vi "TxRx SingleBoard (SubVI).vi"(0 "VISA Refnum in":refnum<visa-resource-name>, 2 "DataMessage Tx":T2={"Send Debug"="", "idx"=0, "DataType"=enum."Int", "Cmd id"=200, "Get/Set"=enum."Set"}, 3 "Tx":refnum<vi>, 4 "Rx":refnum<vi>, 5 "error in (no error)":errorcluster, 6 "Tx semaphore":T1, 8 "Rx semaphore":T1) -> (12 "output array":u8[](array[numeric]) format="%.0x", 14 "VISA Refnum out":refnum<visa-resource-name>, 15 "RxMessage":u8[](array[numeric]) format="%x", 16 "DataReceived?":bool, 17 "CRC":bool, 18 "Get/Set":enum8{"Set", "Get"}(ring), 19 "error out":errorcluster)   [LabVIEW 2017]
panel:
  out "TxMsg":u8[](array[numeric]) format="%.0x"
  # "Value"
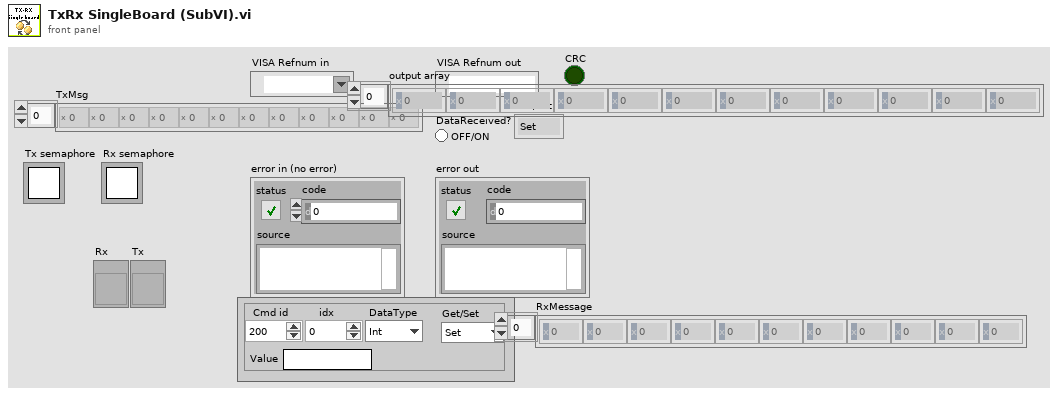
[diagram p1: front panel]
types:
  T1 = typedef "Semaphore RefNum" = refnum<k1>
  T2 = cluster{"Send Debug":string, "idx":u16, "DataType":enum8{"Int", " float"}, "Cmd id":u16, "Get/Set":enum8{"Set", "Get"}}
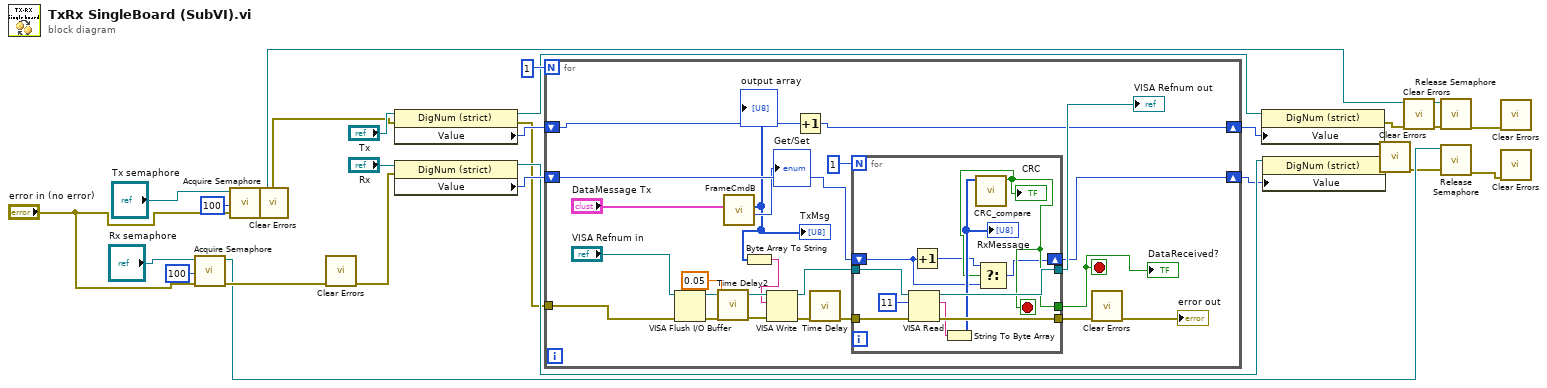
[diagram p0: block diagram]
diagram:
  n1 = call <vilib>:"Acquire Semaphore.vi"("error in (no error)"="error in (no error)", "ms timeout (-1)"=100, "semaphore"="Rx semaphore") -> ("error out"=w12:errorcluster, "semaphore out"=w8:T1)  [unwired: 2 in, 1 out]
  n2 = call <vilib>:"Acquire Semaphore.vi"("error in (no error)"="error in (no error)", "ms timeout (-1)"=100, "semaphore"="Tx semaphore") -> ("error out"=w16:errorcluster, "semaphore out"=w11:T1)  [unwired: 2 in, 1 out]
  n3 = call <vilib>:"Clear Errors.vi"("error in (no error)"=w16) -> ("error out"=w2:errorcluster)  [unwired: 5 in, 1 out]
  n4 = call <vilib>:"Clear Errors.vi"("error in (no error)"=w12) -> ("error out"=w1:errorcluster)  [unwired: 5 in, 1 out]
  n5 = property class="DigNum (strict)"(reference="Tx", error in=w2) -> (reference out=w22:refnum<vi>, error out=w15:errorcluster, "Value"=w23:u64)
  n6 = property class="DigNum (strict)"(reference="Rx", error in=w1) -> (reference out=w21:refnum<vi>, "Value"=w24:u64)  [unwired: 1 out]
  n7 = for {
    N: 1 -> [_]
    shift-right: [w36] -> w20
    shift-left: w23 -> [w38]
    shift-right: [w35] -> w19
    shift-left: w24 -> [w37]
    tunnel: w15 -> [w34]
    stop <- w41 stop-if-true
    n8 = VISA Flush I/O Buffer(VISA resource name="VISA Refnum in", error in (no error)=w34) -> (VISA resource name out=w44:refnum<visa-resource-name>, error out=w33:errorcluster)  [unwired: 1 in]
    n9 = call "Time Delay2"("error in (no error)"=w33, "Delay Time (s)"=0.05) -> ("error out"=w32:errorcluster)  [unwired: 9 in]
    n10 = call "FrameCmdB.vi"("DataMessage"="DataMessage Tx") -> ("Get/Set"=→"Get/Set":enum8{"Set", "Get"}, "output array"=w29:u8[])  [unwired: 7 in, 2 out]
    "TxMsg" <- w29
    "output array" <- w29
    n11 = Byte Array To String(unsigned byte array=w29) -> (string=w28:string)
    n12 = VISA Write(VISA resource name=w44, write buffer=w28, error in (no error)=w32) -> (VISA resource name out=w45:refnum<visa-resource-name>, error out=w48:errorcluster)  [unwired: 1 out]
    n13 = Increment(x=w38) -> (x+1=w36:u64)
    n14 = call "Time Delay"("error in (no error)"=w48) -> ("error out"=w49:errorcluster)  [unwired: 10 in]
    n15 = for {
      N: 1 -> [_]
      tunnel: [w53] -> w41
      tunnel: w49 -> [w60]
      tunnel: [w58] -> w46
      tunnel: w45 -> [w56]
      tunnel: [w59] -> w47
      shift-right: [w50] -> w35
      shift-left: w37 -> [w51]
      stop <- w53 stop-if-true
      n16 = VISA Read(VISA resource name=w56, byte count=u32 11, error in (no error)=w60) -> (VISA resource name out=w59:refnum<visa-resource-name>, read buffer=w55:string, error out=w58:errorcluster)  [unwired: 1 out]
      n17 = Increment(x=w51) -> (x+1=w52:u64)
      n18 = String To Byte Array(string=w55) -> (unsigned byte array=w54:u8[])
      "RxMessage" <- w54
      n19 = call "CRC_compare.vi"("array_in"=w54) -> ("CRC"=w53:bool)  [unwired: 7 in, 3 out]
      "CRC" <- w53
      n20 = Select(t=w52, s=w53, f=w51) -> (s? t:f=w50:u64)
    }
    "DataReceived?" <- w41
    "VISA Refnum out" <- w47
    n21 = call <vilib>:"Clear Errors.vi"("error in (no error)"=w46) -> ("error out"=→"error out":errorcluster)  [unwired: 5 in, 1 out]
  }
  n22 = property class="DigNum (strict)"(reference=w22, "Value"=w20) -> (error out=w10:errorcluster)  [unwired: 1 in, 1 out]
  n23 = property class="DigNum (strict)"(reference=w21, "Value"=w19) -> (error out=w9:errorcluster)  [unwired: 1 in, 1 out]
  n24 = call <vilib>:"Clear Errors.vi"("error in (no error)"=w9) -> ("error out"=w5:errorcluster)  [unwired: 5 in, 1 out]
  n25 = call <vilib>:"Clear Errors.vi"("error in (no error)"=w10) -> ("error out"=w6:errorcluster)  [unwired: 5 in, 1 out]
  n26 = call <vilib>:"Release Semaphore.vi"("error in (no error)"=w6, "semaphore"=w11) -> ("error out"=w4:errorcluster)  [unwired: 4 in, 1 out]
  n27 = call <vilib>:"Release Semaphore.vi"("error in (no error)"=w5, "semaphore"=w8) -> ("error out"=w3:errorcluster)  [unwired: 4 in, 1 out]
  n28 = call <vilib>:"Clear Errors.vi"("error in (no error)"=w4) -> ()  [unwired: 5 in, 2 out]
  n29 = call <vilib>:"Clear Errors.vi"("error in (no error)"=w3) -> ()  [unwired: 5 in, 2 out]
